vi "Keith 7001 Display Message.vi"(1 "bottom display message":string="HI BOB", 2 "bottom enable/disable":bool, 3 "status messages":bool, 4 "error in":T1, 5 "top display message":string="HI BOB", 6 "top enable/disable":bool, 7 "GPIB address":string="7") -> (0 "error out":T1)   [LabVIEW 2019]
doc: "This VI for the Keithley 7001 Switch System allows the operator to set two user defined messages on the front panel of the instrument. The top message can be up to 20 characters and the bottom message can be up to 32 characters. This VI also allows the operator to enable/disable the unit's status messages."
panel:
  # "enable\ndisable"
  # "enable\ndisable"
  # "enable\ndisable"
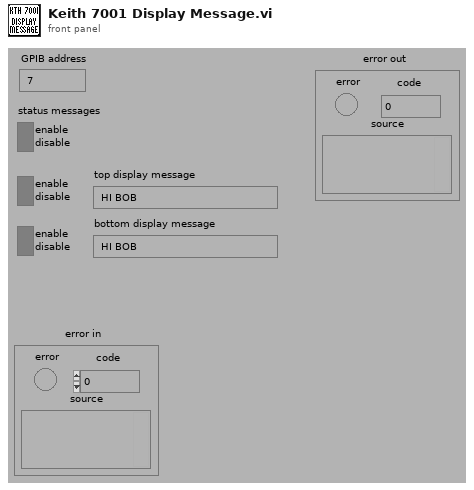
[diagram p1: front panel]
types:
  T1 = cluster{"error":bool, "code":i32, "source":string}
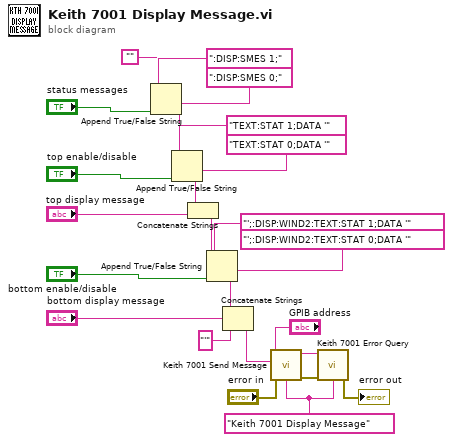
[diagram p0: block diagram]
diagram:
  w2 = "Keith 7001 Display Message"
  n1 = Append True/False String(1:"status messages", 2:":DISP:SMES 0;", 3:":DISP:SMES 1;", 4:"") -> (0:w9:string)
  n2 = Append True/False String(1:"top enable/disable", 2:"TEXT:STAT 0;DATA '", 3:"TEXT:STAT 1;DATA '", 4:w9) -> (0:w11:string)
  n3 = Concatenate Strings(w11, "top display message") -> (w20:string)
  n4 = Append True/False String(1:"bottom enable/disable", 2:"';:DISP:WIND2:TEXT:STAT 0;DATA '", 3:"';:DISP:WIND2:TEXT:STAT 1;DATA '", 4:w20) -> (0:w19:string)
  n5 = Concatenate Strings(w19, "bottom display message", "'") -> (w17:string)
  n6 = call "Keith 7001 Send Message.vi"("address string"="GPIB address", "write buffer"=w17, "source"=w2, "error in"="error in") -> ("address out"=w4:string, "error out"=w3:T1)  [unwired: 2 in, 2 out]
  n7 = call "Keith 7001 Error Query.vi"("GPIB address"=w4, "error in"=w3, "source"=w2) -> ("error out"=→"error out":T1)  [unwired: 2 out]
